vi "OBD Get Parameters.vi"(7 "Error In":errorcluster, 9 "Supported PIDs":u8[](array[numeric])=[1, 3, 4, 5, 6, 7, 12, 13, 14, 15, 16, 17, 18, 19, 21, 28, 31, 32, 33, 46, 47, 48, 49, 51, 52, 60, 64, 65, 66, 67, 68, 69, 70, 71, 73, 74, 76] format="%x", 10 "diag ref in":T2={"Diag CAN Handle"=0, "Transport Protocol"=enum."ISO TP - Normal Mode", "Receive Address Extension"=0, "Transmit Address Extension"=0, "Receive CAN Id"=0, "Transmit CAN Id"=0, "Log Frames ?"=FALSE, "My TP Address"=0, "Other TP Address"=0, "T1"=0, "T2"=0, "T3"=0, "T4"=0, "Tx SN"=0, "Block Size"=0, "Rx SN"=0, "VW TP Initialized?"=FALSE, "Tx block no"=0, "baud rate"=0, "Interface"="", "Channel Diag CAN Handle"=0, "UDP Connection ID"=refnum, "TCP Connection ID"=refnum, "Target IP Addr"=0, "Source Address"=0, "Target Address"=0, "Send Header NACK?"=FALSE, "DLL Handle"=0, "NAD"=0, "Time Stamp read first"=0.0, "Time Stamp read last"=0.0, "Time Stamp write first"=0.0, "Time Stamp write last"=0.0, "Time Stamp write"=0.0, "Time Stamp read"=0.0, " I/O Mode"=0, "FD Baudrate"=0, "TX_DL"=8, "RX_DL"=8, "DoIP Protocol Version"=1, " Selected I/O Mode"=0, "TesterPresent Counter"=0, "TesterPresent Limit"=0, "TesterPresent Tick[ms]"=10, "TesterPresent RequireResponse?"=FALSE, "TesterPresent Stored Ref?"=FALSE, "TesterPresent Message"=[], "TesterPresent Task Handle"=0, "TesterPresent Semaphore"=refnum, "Response Plausibility Check"=1, "Default Version?"=TRUE, "Diagostic Globals"={"Timeout FC (Bs)"=250, "Timeout CF (Cr)"=250, "Timeout Diag Command"=1000, "Receive Block Size (BS)"=0, "Wait Time CF (STmin)"=5, "Max Waits (N_WFTmax)"=10, "Waits to Send (N_WAIT)"=0, "Time between Waits (TW)"=25, "Fill CAN Frames?"=TRUE, "Fill Byte"=255, "Invalid Response as Error?"=FALSE, "Max RspPending Count"=5, "VWTP Command Timeout"=50, "Transport Protocol"=enum."Diagnostics on IP", "Diag CAN Handle"=0, "DLL Handle"=0, "Timeout RspPending"=1000}, "Session-based Properties?"=FALSE} {"Diagostic Globals"."Fill Byte" format="%x"; "TesterPresent Message" format="%.0x"; "Selected I/O Mode" items=["CAN", "CAN FD", "CAN FD+BRS", "ECU Determined"]; "DoIP Protocol Version" items=["2010"=1, "2012"=2]; "RX_DL" items=["8"=8, "12"=12, "16"=16, "20"=20, "24"=24, "32"=32, "48"=48, "64"=64]; "TX_DL" items=["8"=8, "12"=12, "16"=16, "20"=20, "24"=24, "32"=32, "48"=48, "64"=64]; "I/O Mode" items=["CAN", "CAN FD", "CAN FD+BRS", "Not yet determined"]}) -> (0 "error out":errorcluster, 2 "Diagnostic Data":T1 {"OBD Compliance Level" items=["(error)", "OBD II (California ARB)", "OBD (Federal EPA)", "OBD and OBD II", "OBD I", "Not OBD Compliant", "EOBD", "EBOD and OBD II", "EOBD and OBD", "EOBD, OBD, and OBDII", "JOBD", "JOBD and OBD II", "JOBD and EOBD", "JOBD, EOBD, and OBD II"]; "MIL Lamp" format="%.0x"}, 3 "diag ref out":T2={"Diag CAN Handle"=0, "Transport Protocol"=enum."ISO TP - Normal Mode", "Receive Address Extension"=0, "Transmit Address Extension"=0, "Receive CAN Id"=0, "Transmit CAN Id"=0, "Log Frames ?"=FALSE, "My TP Address"=0, "Other TP Address"=0, "T1"=0, "T2"=0, "T3"=0, "T4"=0, "Tx SN"=0, "Block Size"=0, "Rx SN"=0, "VW TP Initialized?"=FALSE, "Tx block no"=0, "baud rate"=0, "Interface"="", "Channel Diag CAN Handle"=0, "UDP Connection ID"=refnum, "TCP Connection ID"=refnum, "Target IP Addr"=0, "Source Address"=0, "Target Address"=0, "Send Header NACK?"=FALSE, "DLL Handle"=0, "NAD"=0, "Time Stamp read first"=0.0, "Time Stamp read last"=0.0, "Time Stamp write first"=0.0, "Time Stamp write last"=0.0, "Time Stamp write"=0.0, "Time Stamp read"=0.0, " I/O Mode"=0, "FD Baudrate"=0, "TX_DL"=8, "RX_DL"=8, "DoIP Protocol Version"=1, " Selected I/O Mode"=0, "TesterPresent Counter"=0, "TesterPresent Limit"=0, "TesterPresent Tick[ms]"=10, "TesterPresent RequireResponse?"=FALSE, "TesterPresent Stored Ref?"=FALSE, "TesterPresent Message"=[], "TesterPresent Task Handle"=0, "TesterPresent Semaphore"=refnum, "Response Plausibility Check"=1, "Default Version?"=TRUE, "Diagostic Globals"={"Timeout FC (Bs)"=250, "Timeout CF (Cr)"=250, "Timeout Diag Command"=1000, "Receive Block Size (BS)"=0, "Wait Time CF (STmin)"=5, "Max Waits (N_WFTmax)"=10, "Waits to Send (N_WAIT)"=0, "Time between Waits (TW)"=25, "Fill CAN Frames?"=TRUE, "Fill Byte"=255, "Invalid Response as Error?"=FALSE, "Max RspPending Count"=5, "VWTP Command Timeout"=50, "Transport Protocol"=enum."Diagnostics on IP", "Diag CAN Handle"=0, "DLL Handle"=0, "Timeout RspPending"=1000}, "Session-based Properties?"=FALSE} {"Diagostic Globals"."Fill Byte" format="%x"; "TesterPresent Message" format="%.0x"; "Selected I/O Mode" items=["CAN", "CAN FD", "CAN FD+BRS", "ECU Determined"]; "DoIP Protocol Version" items=["2010"=1, "2012"=2]; "RX_DL" items=["8"=8, "12"=12, "16"=16, "20"=20, "24"=24, "32"=32, "48"=48, "64"=64]; "TX_DL" items=["8"=8, "12"=12, "16"=16, "20"=20, "24"=24, "32"=32, "48"=48, "64"=64]; "I/O Mode" items=["CAN", "CAN FD", "CAN FD+BRS", "Not yet determined"]})   [LabVIEW 2018]
uses:
  <vilib>/Automotive Diagnostic Command Set/Diagnostic Transport.llb/Diag Reference.ctl
  <vilib>/Automotive Diagnostic Command Set/Diagnostic Transport.llb/Transport Protocol Selector.ctl
  <vilib>/Automotive Diagnostic Command Set/Diagnostic Transport.llb/DoIP Protocol Version.ctl
  <vilib>/Automotive Diagnostic Command Set/Diagnostic Transport.llb/Diag Globals.ctl
  OBD Data Typedef.ctl
  OBD_Compliance.vi
  OBD_MIL_Lamp.vi
  OBD_Engine_RPM.vi
  OBD_Current_Throttle Position.vi
  OBD_MAF_Airflow_Rate.vi
  OBD_Vehicle Speed.vi
  OBD_Timing Advance.vi
  OBD_Intake_Air_Temp.vi
  OBD_Engine Coolant Temp.vi
  OBD_Calculated Load Value.vi
  OBD_Time Since Engine Start.vi
  <vilib>/addons/Automotive Diagnostic Command Set/NI_Automotive Diagnostic Command Set.lvlib
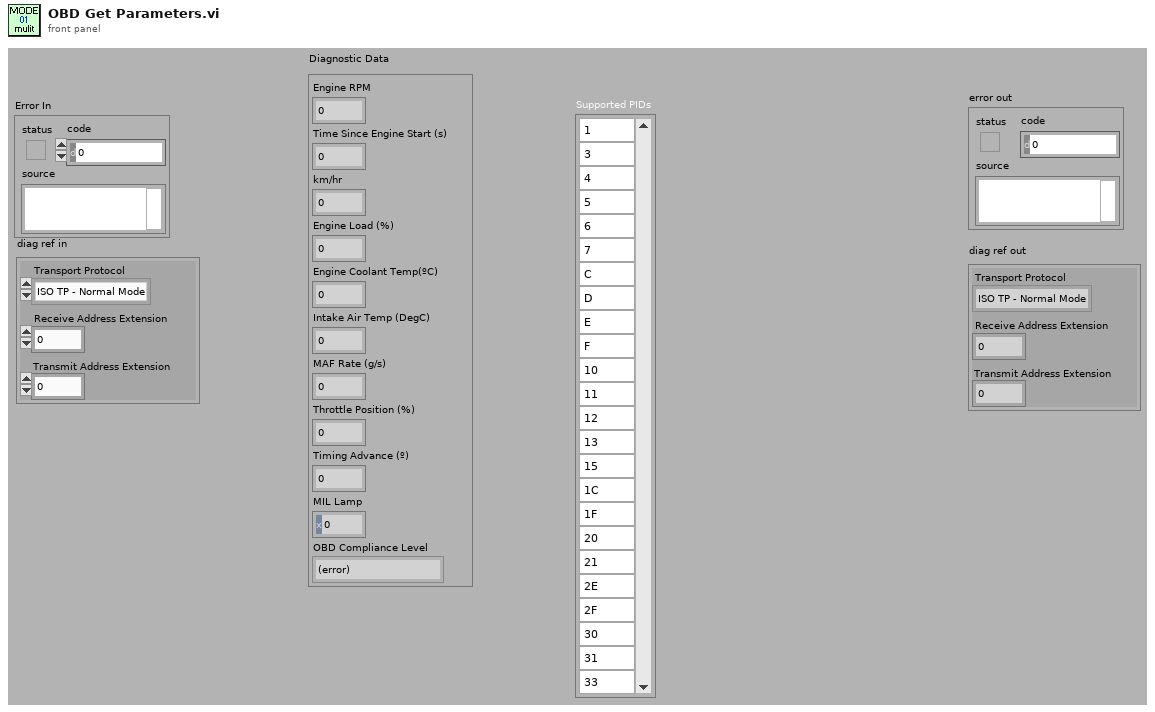
[diagram p1: front panel]
types:
  T1 = typedef "OBD Data Typedef.ctl" = cluster{"Engine RPM":dbl, "Time Since Engine Start (s)":dbl, "km/hr":dbl, "Engine Load (%)":dbl, "Engine Coolant Temp(ºC)":dbl, "Intake Air Temp (DegC)":dbl, "MAF Rate (g/s)":dbl, "Throttle Position (%)":dbl, "Timing Advance (º)":dbl, "MIL Lamp":u32, "OBD Compliance Level":u16}
  T2 = typedef "NI_Automotive Diagnostic Command Set.lvlib/Diag Reference.ctl" = cluster{"Diag CAN Handle":u32, "Transport Protocol":T3, "Receive Address Extension":u8, "Transmit Address Extension":u8, "Receive CAN Id":u32, "Transmit CAN Id":u32, "Log Frames ?":bool, "My TP Address":u8, "Other TP Address":u8, "T1":u16, "T2":u16, "T3":u16, "T4":u16, "Tx SN":u8, "Block Size":u8, "Rx SN":u8, "VW TP Initialized?":bool, "Tx block no":u8, "baud rate":u64, "Interface":string, "Channel Diag CAN Handle":u32, "UDP Connection ID":refnum<k16>, "TCP Connection ID":refnum<k5>, "Target IP Addr":u32, "Source Address":u16, "Target Address":u16, "Send Header NACK?":bool, "DLL Handle":u32, "NAD":u8, "Time Stamp read first":dbl, "Time Stamp read last":dbl, "Time Stamp write first":dbl, "Time Stamp write last":dbl, "Time Stamp write":dbl, "Time Stamp read":dbl, " I/O Mode":u32, "FD Baudrate":u64, "TX_DL":u16, "RX_DL":u16, "DoIP Protocol Version":T4, " Selected I/O Mode":u32, "TesterPresent Counter":u32, "TesterPresent Limit":u32, "TesterPresent Tick[ms]":i32, "TesterPresent RequireResponse?":bool, "TesterPresent Stored Ref?":bool, "TesterPresent Message":u8[], "TesterPresent Task Handle":i32, "TesterPresent Semaphore":T5, "Response Plausibility Check":u32, "Default Version?":bool, "Diagostic Globals":T6, "Session-based Properties?":bool}
  T3 = typedef "NI_Automotive Diagnostic Command Set.lvlib/Transport Protocol Selector.ctl" = enum16{"ISO TP - Normal Mode", "ISO TP - Mixed Mode", "VW TP 2.0", "Diagnostics on IP", "ISO TP LIN"}
  T4 = typedef "NI_Automotive Diagnostic Command Set.lvlib/DoIP Protocol Version.ctl" = u8
  T5 = typedef "Semaphore RefNum" = refnum<k1>
  T6 = typedef "NI_Automotive Diagnostic Command Set.lvlib/Diag Globals.ctl" = cluster{"Timeout FC (Bs)":u32, "Timeout CF (Cr)":u32, "Timeout Diag Command":u32, "Receive Block Size (BS)":u8, "Wait Time CF (STmin)":u8, "Max Waits (N_WFTmax)":u8, "Waits to Send (N_WAIT)":i32, "Time between Waits (TW)":u32, "Fill CAN Frames?":bool, "Fill Byte":u32, "Invalid Response as Error?":bool, "Max RspPending Count":u32, "VWTP Command Timeout":u32, "Transport Protocol":T3, "Diag CAN Handle":u32, "DLL Handle":u32, "Timeout RspPending":u32}
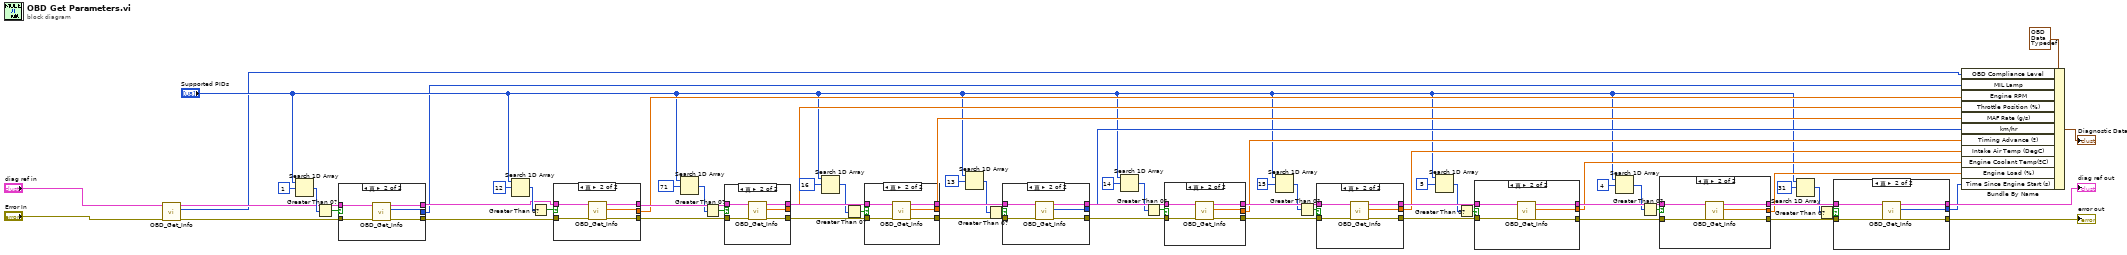
[diagram p0: block diagram]
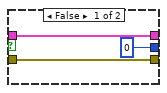
[diagram p2: hidden frame]
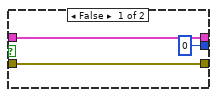
[diagram p3: hidden frame]
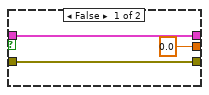
[diagram p4: hidden frame]
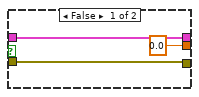
[diagram p5: hidden frame]
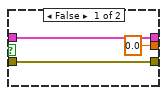
[diagram p6: hidden frame]
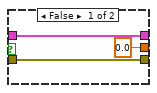
[diagram p7: hidden frame]
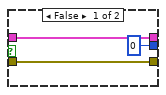
[diagram p8: hidden frame]
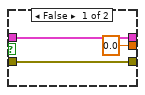
[diagram p9: hidden frame]
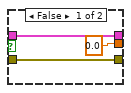
[diagram p10: hidden frame]
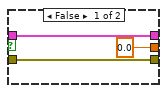
[diagram p11: hidden frame]
diagram:
  n1 = call-poly "OBD_Get_Info.vi"("error in (no error)"="Error In", "diag ref in"="diag ref in") -> ("error out"=w2:errorcluster, "OBD Compliance Level"=w1:u16, "diag ref out"=w3:T2)  [unwired: 7 in]
  n2 = Search 1D Array(1D array="Supported PIDs", element=u8 1) -> (index of element=w12:i32)  [unwired: 1 in]
  n3 = Greater Than 0?(x=w12) -> (x > 0?=w13:bool)
  n4 = case shown="真" w13 {
    tunnel: w3 -> [w71 w76]
    tunnel: [w70 w75] -> w10
    tunnel: w2 -> [w70 w74]
    tunnel: [w71 w73] -> w9
    tunnel: [u32 0 ("Engine RPM") w72] -> w6
    frame False {
    }
    frame True {
      n5 = call-poly "OBD_Get_Info.vi"("error in (no error)"=w74, "diag ref in"=w76) -> ("error out"=w75:errorcluster, "Engine RPM"=w72:u32, "diag ref out"=w73:T2)  [unwired: 7 in]
    }
  }
  n6 = Search 1D Array(1D array="Supported PIDs", element=u8 12) -> (index of element=w39:i32)  [unwired: 1 in]
  n7 = Greater Than 0?(x=w39) -> (x > 0?=w38:bool)
  n8 = case shown="真" w38 {
    tunnel: w9 -> [w79 w84]
    tunnel: [w78 w83] -> w53
    tunnel: w10 -> [w78 w82]
    tunnel: [w79 w81] -> w51
    tunnel: [0.0 ("Engine RPM") w80] -> w50
    frame False {
    }
    frame True {
      n9 = call-poly "OBD_Get_Info.vi"("error in (no error)"=w82, "diag ref in"=w84) -> ("error out"=w83:errorcluster, "Engine RPM"=w80:dbl, "diag ref out"=w81:T2)  [unwired: 7 in]
    }
  }
  n10 = Search 1D Array(1D array="Supported PIDs", element=u8 71) -> (index of element=w36:i32)  [unwired: 1 in]
  n11 = Greater Than 0?(x=w36) -> (x > 0?=w35:bool)
  n12 = case shown="真" w35 {
    tunnel: [w86 w92] -> w54
    tunnel: w53 -> [w86 w91]
    tunnel: [w87 w90] -> w52
    tunnel: w51 -> [w87 w89]
    tunnel: [0.0 ("Throttle Position (%)") w88] -> w49
    frame False {
    }
    frame True {
      n13 = call-poly "OBD_Get_Info.vi"("error in (no error)"=w91, "diag ref in"=w89) -> ("error out"=w92:errorcluster, "Throttle Position (%)"=w88:dbl, "diag ref out"=w90:T2)  [unwired: 7 in]
    }
  }
  n14 = Search 1D Array(1D array="Supported PIDs", element=u8 16) -> (index of element=w32:i32)  [unwired: 1 in]
  n15 = Greater Than 0?(x=w32) -> (x > 0?=w33:bool)
  n16 = case shown="真" w33 {
    tunnel: [w94 w100] -> w56
    tunnel: [w95 w99] -> w55
    tunnel: w54 -> [w94 w98]
    tunnel: w52 -> [w95 w97]
    tunnel: [0.0 ("MAF Rate (g/s)") w96] -> w48
    frame False {
    }
    frame True {
      n17 = call-poly "OBD_Get_Info.vi"("error in (no error)"=w98, "diag ref in"=w97) -> ("error out"=w100:errorcluster, "MAF Rate (g/s)"=w96:dbl, "diag ref out"=w99:T2)  [unwired: 7 in]
    }
  }
  n18 = Search 1D Array(1D array="Supported PIDs", element=u8 13) -> (index of element=w30:i32)  [unwired: 1 in]
  n19 = Greater Than 0?(x=w30) -> (x > 0?=w29:bool)
  n20 = case shown="真" w29 {
    tunnel: [w102 w108] -> w58
    tunnel: [w103 w107] -> w57
    tunnel: w56 -> [w102 w106]
    tunnel: w55 -> [w103 w105]
    tunnel: [u8 0 ("km/hr") w104] -> w47
    frame False {
    }
    frame True {
      n21 = call-poly "OBD_Get_Info.vi"("error in (no error)"=w106, "diag ref in"=w105) -> ("error out"=w108:errorcluster, "km/hr"=w104:u8, "diag ref out"=w107:T2)  [unwired: 7 in]
    }
  }
  n22 = Search 1D Array(1D array="Supported PIDs", element=u8 14) -> (index of element=w26:i32)  [unwired: 1 in]
  n23 = Greater Than 0?(x=w26) -> (x > 0?=w27:bool)
  n24 = case shown="真" w27 {
    tunnel: [w110 w116] -> w60
    tunnel: [w111 w115] -> w59
    tunnel: w58 -> [w110 w114]
    tunnel: w57 -> [w111 w113]
    tunnel: [0.0 ("Timing Advance (º)") w112] -> w46
    frame False {
    }
    frame True {
      n25 = call-poly "OBD_Get_Info.vi"("error in (no error)"=w114, "diag ref in"=w113) -> ("error out"=w116:errorcluster, "Timing Advance (º)"=w112:dbl, "diag ref out"=w115:T2)  [unwired: 7 in]
    }
  }
  n26 = Search 1D Array(1D array="Supported PIDs", element=u8 15) -> (index of element=w23:i32)  [unwired: 1 in]
  n27 = Greater Than 0?(x=w23) -> (x > 0?=w24:bool)
  n28 = case shown="真" w24 {
    tunnel: [w119 w124] -> w62
    tunnel: [w118 w123] -> w61
    tunnel: w60 -> [w118 w122]
    tunnel: w59 -> [w119 w121]
    tunnel: [0.0 ("Intake Air Temp (DegC)") w120] -> w44
    frame False {
    }
    frame True {
      n29 = call-poly "OBD_Get_Info.vi"("error in (no error)"=w122, "diag ref in"=w121) -> ("error out"=w123:errorcluster, "Intake Air Temp (DegC)"=w120:dbl, "diag ref out"=w124:T2)  [unwired: 7 in]
    }
  }
  n30 = Search 1D Array(1D array="Supported PIDs", element=u8 5) -> (index of element=w20:i32)  [unwired: 1 in]
  n31 = Greater Than 0?(x=w20) -> (x > 0?=w21:bool)
  n32 = case shown="真" w21 {
    tunnel: [w127 w132] -> w64
    tunnel: [w126 w131] -> w63
    tunnel: w62 -> [w127 w130]
    tunnel: w61 -> [w126 w129]
    tunnel: [0.0 ("Engine Coolant Temp(ºC)") w128] -> w43
    frame False {
    }
    frame True {
      n33 = call-poly "OBD_Get_Info.vi"("error in (no error)"=w129, "diag ref in"=w130) -> ("error out"=w131:errorcluster, "Engine Coolant Temp(ºC)"=w128:dbl, "diag ref out"=w132:T2)  [unwired: 7 in]
    }
  }
  n34 = Search 1D Array(1D array="Supported PIDs", element=u8 4) -> (index of element=w17:i32)  [unwired: 1 in]
  n35 = Greater Than 0?(x=w17) -> (x > 0?=w18:bool)
  n36 = case shown="真" w18 {
    tunnel: [w135 w140] -> w66
    tunnel: [w134 w139] -> w65
    tunnel: w64 -> [w135 w138]
    tunnel: w63 -> [w134 w137]
    tunnel: [0.0 ("Engine Load (%)") w136] -> w42
    frame False {
    }
    frame True {
      n37 = call-poly "OBD_Get_Info.vi"("error in (no error)"=w137, "diag ref in"=w138) -> ("error out"=w139:errorcluster, "Engine Load (%)"=w136:dbl, "diag ref out"=w140:T2)  [unwired: 7 in]
    }
  }
  n38 = Search 1D Array(1D array="Supported PIDs", element=u8 31) -> (index of element=w14:i32)  [unwired: 1 in]
  n39 = Greater Than 0?(x=w14) -> (x > 0?=w15:bool)
  n40 = case shown="真" w15 {
    tunnel: [w142 w148] -> w68
    tunnel: [w143 w147] -> w67
    tunnel: w66 -> [w143 w146]
    tunnel: w65 -> [w142 w145]
    tunnel: [u16 0 ("Time Since Engine Start (s)") w144] -> w41
    frame False {
    }
    frame True {
      n41 = call-poly "OBD_Get_Info.vi"("error in (no error)"=w145, "diag ref in"=w146) -> ("error out"=w148:errorcluster, "Time Since Engine Start (s)"=w144:u16, "diag ref out"=w147:T2)  [unwired: 7 in]
    }
  }
  "error out" <- w68
  "diag ref out" <- w67
  n42 = Bundle By Name(cluster=T1 {"Engine RPM"=0.0, "Time Since Engine Start (s)"=0.0, "km/hr"=0.0, "Engine Load (%)"=0.0, "Engine Coolant Temp(ºC)"=0.0, "Intake Air Temp (DegC)"=0.0, "MAF Rate (g/s)"=0.0, "Throttle Position (%)"=0.0, "Timing Advance (º)"=0.0, "MIL Lamp"=0, "OBD Compliance Level"=0} ("Diagnostic Data 2"), "OBD Compliance Level"=w1, "MIL Lamp"=w6, "Engine RPM"=w50, "Throttle Position (%)"=w49, "MAF Rate (g/s)"=w48, "km/hr"=w47, "Timing Advance (º)"=w46, "Intake Air Temp (DegC)"=w44, "Engine Coolant Temp(ºC)"=w43, "Engine Load (%)"=w42, "Time Since Engine Start (s)"=w41) -> (→"Diagnostic Data":T1)
